vi "handler.vi"(10 "exec queue":refnum<queue>, 11 "connection":refnum<k5>) -> ()   [LabVIEW 2013]
uses:
  worker package.ctl
  application request.ctl
  begin request role.ctl
  record header.ctl
  record types.ctl
  end request body.ctl
  end request protocol status.ctl
  begin request body.ctl
  parse record header.vi
  parse count.vi
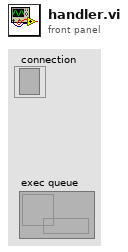
[diagram p1: front panel]
types:
  T1 = typedef "record types.ctl" = enum8{"Error", "Begin Request", "Abort Request", "End Request", "Parameters", "Standard Input", "Standard Output", "Standard Error", "Data", "Get Values", "Get Values Result", "Unknown Type"}
  T2 = typedef "record header.ctl" = cluster{"version":u8, "type":T1, "request id":u16, "content length":u16, "padding length":u8, "reserved":u8}
  T3 = typedef "end request protocol status.ctl" = enum8{"complete", "cant mpx connection", "overloaded", "unknown role"}
  T4 = typedef "end request body.ctl" = cluster{"application status":u32, "protocol status":T3, "reserved 1":u8, "reserved 2":u8, "reserved 3":u8}
  T5 = typedef "begin request body.ctl" = cluster{"role":u16, "flags":u8, "reserved 1":u8, "reserved 2":u8, "reserved 3":u8, "reserved 4":u8, "reserved 5":u8}
  T6 = typedef "application request.ctl" = cluster{"request id":u16, "role":T7, "standard input":string, "data":string, "dictionary":variant, "close after response":bool}
  T7 = typedef "begin request role.ctl" = enum16{"none", "Responder", "Authorizer", "Filter"}
  T8 = typedef "worker package.ctl" = cluster{"TCP Connection":refnum<k5>, "application request":T6}
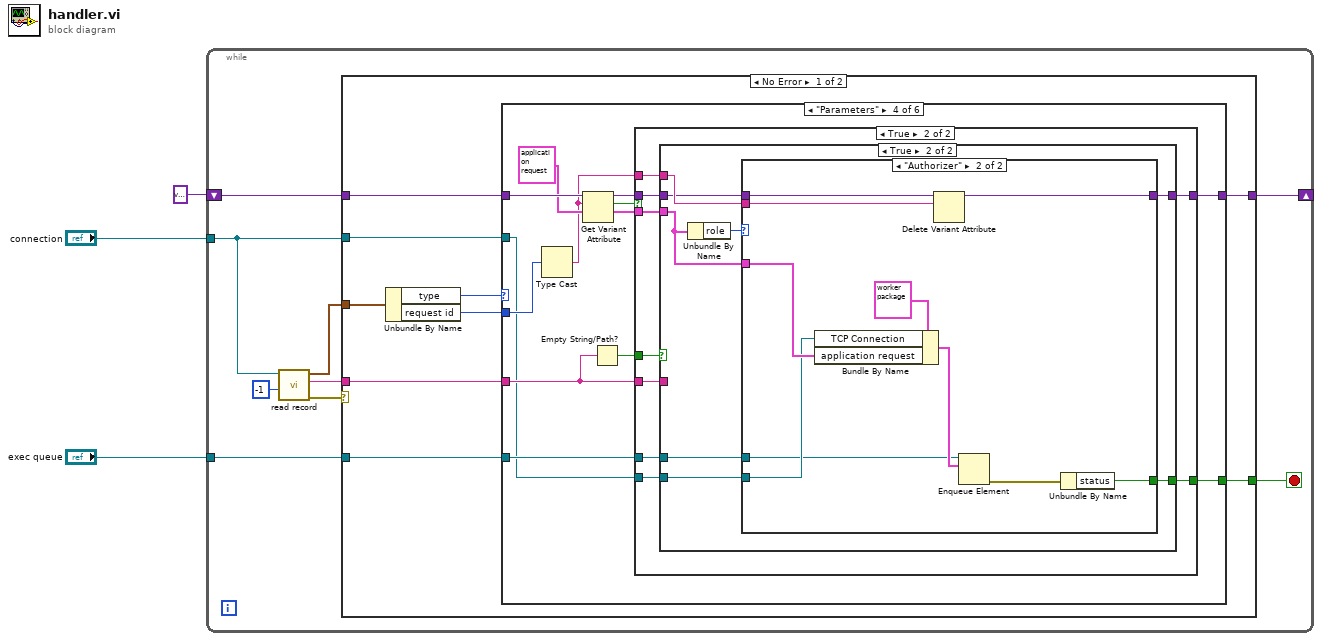
[diagram p0: block diagram]
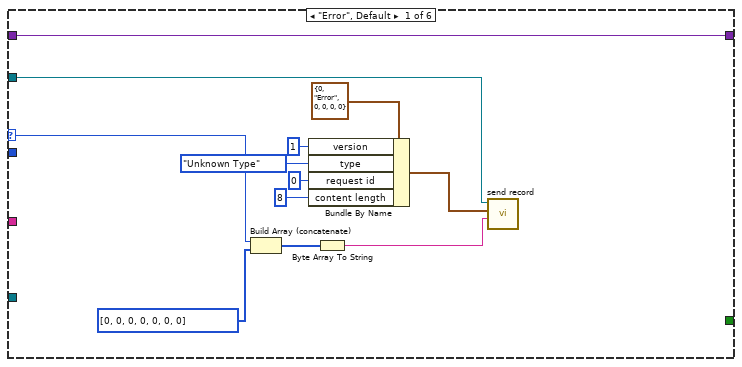
[diagram p2: hidden frame]
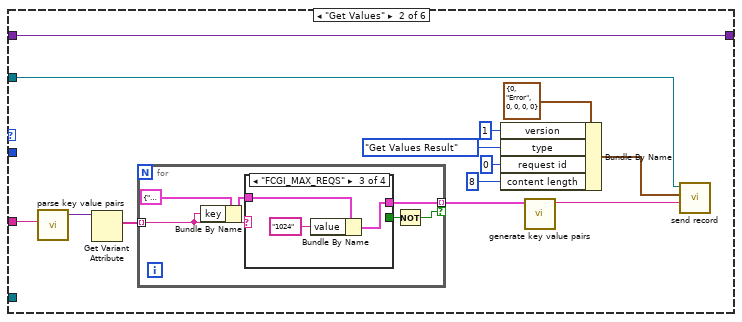
[diagram p3: hidden frame]
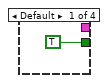
[diagram p4: hidden frame]
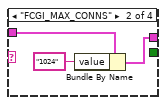
[diagram p5: hidden frame]
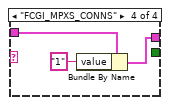
[diagram p6: hidden frame]
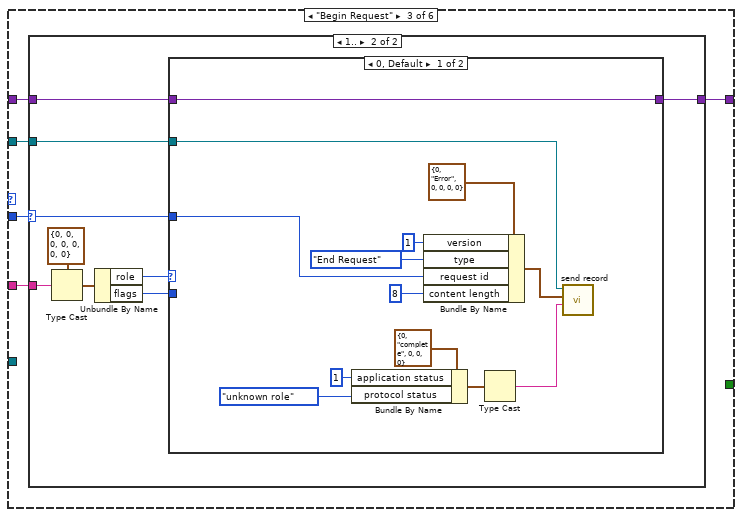
[diagram p7: hidden frame]
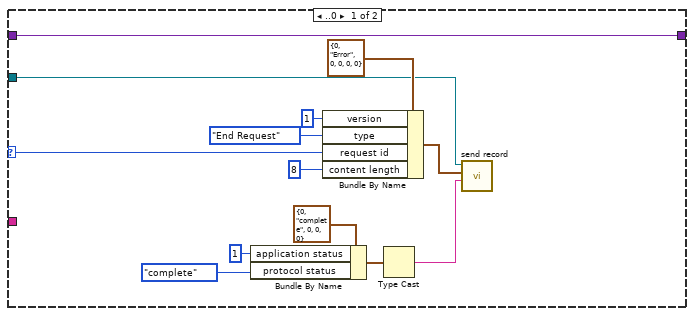
[diagram p8: hidden frame]
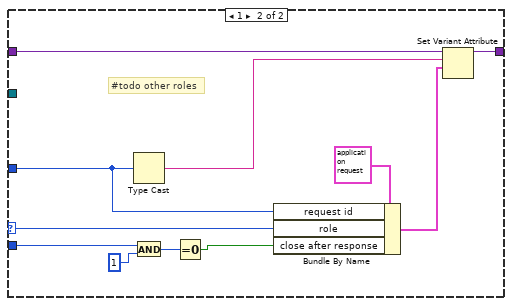
[diagram p9: hidden frame]
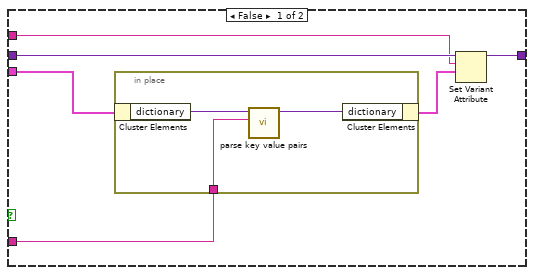
[diagram p11: hidden frame]
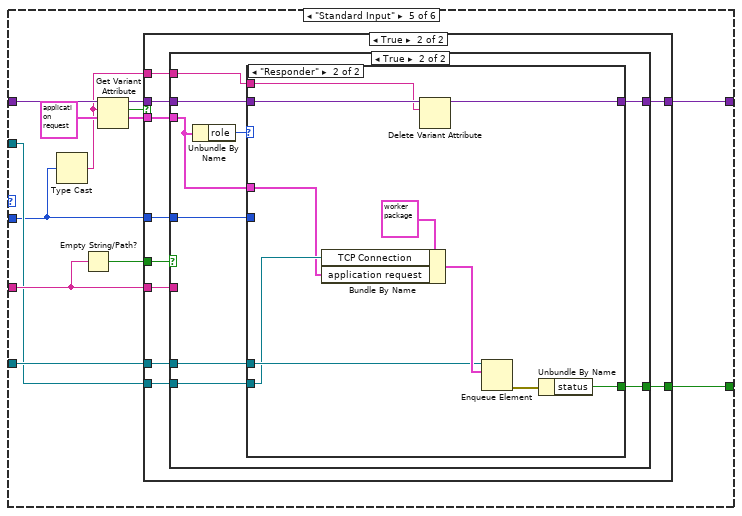
[diagram p13: hidden frame]
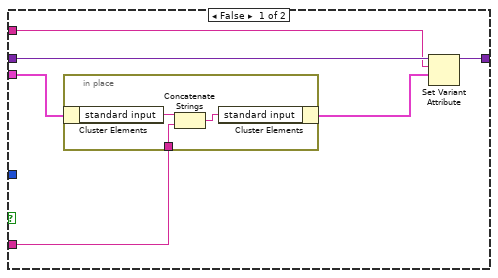
[diagram p15: hidden frame]
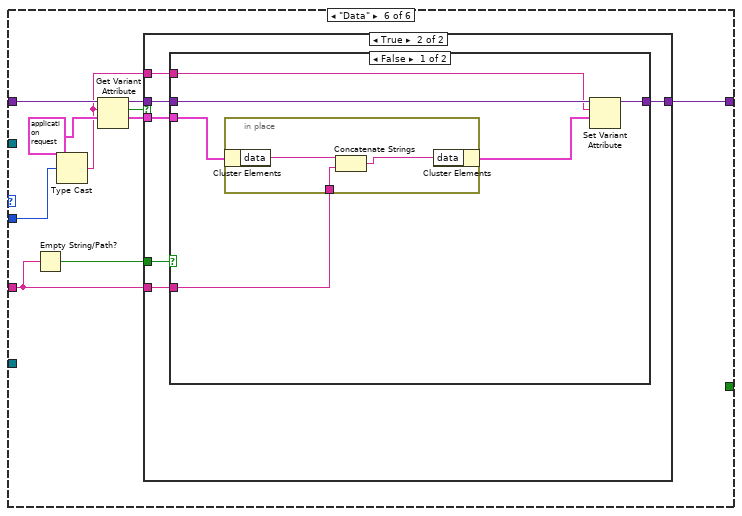
[diagram p17: hidden frame]
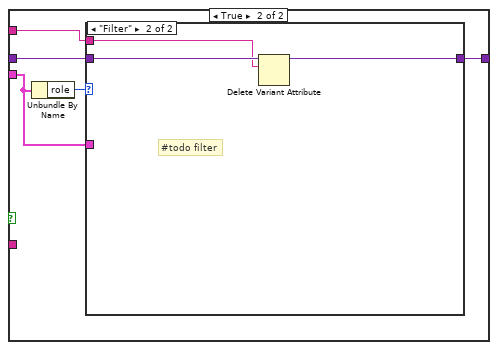
[diagram p19: hidden frame]
diagram:
  n1 = while {
    tunnel: "connection" -> [w6]
    shift-right: [w7] -> _
    shift-left: variant -> [w8]
    tunnel: "exec queue" -> [w4]
    stop <- w5 stop-if-true
    n2 = call "read record.vi"("timeout ms (-1)"=-1, "connection"=w6) -> ("error out"=w11:errorcluster, "data"=w9:string, "header"=w10:T2)  [unwired: 6 in, 1 out]
    n3 = case shown="No Error" w11 {
      tunnel: w10 -> [w21 _]
      tunnel: w9 -> [w15 _]
      tunnel: w8 -> [w19 w254]
      tunnel: [w18 w254] -> w7
      tunnel: w6 -> [w17 _]
      tunnel: [w13 TRUE] -> w5
      tunnel: w4 -> [w14 _]
      frame No Error {
        n4 = Unbundle By Name(w21) -> ("type"=w20:T1, "request id"=w16:u16)
        n5 = case shown="\"Parameters\"" w20 {
          selector: w20 -> [w25 _ _ _ _ _]
          tunnel: w19 -> [w33 w46 w67 w126 w177 w227]
          tunnel: [w33 w46 w65 w125 w176 w226] -> w18
          tunnel: w17 -> [w27 w40 w63 w114 w166 _]
          tunnel: w16 -> [_ _ w64 w124 w165 w225]
          tunnel: w15 -> [_ w36 w66 w123 w175 w224]
          tunnel: w14 -> [_ _ _ w116 w168 _]
          tunnel: [_ _ _ w115 w167 _] -> w13
          frame "Error", Default {
            n6 = Build Array (concatenate)(w25, u8[] [0, 0, 0, 0, 0, 0, 0]) -> (w24:u8[])
            n7 = Bundle By Name(cluster=T2 {"version"=0, "type"=enum."Error", "request id"=0, "content length"=0, "padding length"=0, "reserved"=0} ("header"), "version"=u8 1, "type"=record_types."Unknown Type", "request id"=u16 0, "content length"=u16 8) -> (w26:T2)
            n8 = Byte Array To String(unsigned byte array=w24) -> (string=w23:string)
            n9 = call "send record.vi"("data"=w23, "header"=w26, "connection"=w27) -> ()  [unwired: 8 in, 1 out]
          }
          frame "Get Values" {
            n10 = call "parse key value pairs.vi"("stream"=w36) -> ("dictionary out"=w35:variant)  [unwired: 10 in]
            n11 = Get Variant Attribute(Variant=w35) -> (names=w34:string[])  [unwired: 3 in, 3 out]
            n12 = for {
              tunnel: [w52] -> w37 mode=indexing if=w50
              tunnel: w34 -> [w47] mode=indexing
              n13 = Bundle By Name(cluster=cluster{"key":string, "value":string} {"key"="", "value"=""} ("Cluster"), "key"=w47) -> (w48:cluster{"key":string, "value":string})
              n14 = case shown="\"FCGI_MAX_REQS\"" w47 {
                tunnel: [_ w56 w59 w62] -> w52
                tunnel: [TRUE _ _ _] -> w51
                tunnel: w48 -> [_ w54 w57 w60]
                frame Default {
                }
                frame "FCGI_MAX_CONNS" {
                  n15 = Bundle By Name(cluster=w54, "value"="1024") -> (w56:cluster{"key":string, "value":string})
                }
                frame "FCGI_MAX_REQS" {
                  n16 = Bundle By Name(cluster=w57, "value"="1024") -> (w59:cluster{"key":string, "value":string})
                }
                frame "FCGI_MPXS_CONNS" {
                  n17 = Bundle By Name(cluster=w60, "value"="1") -> (w62:cluster{"key":string, "value":string})
                }
              }
              n18 = Not(x=w51) -> (.not. x?=w50:bool)
            }
            n19 = Bundle By Name(cluster=T2 {"version"=0, "type"=enum."Error", "request id"=0, "content length"=0, "padding length"=0, "reserved"=0} ("header"), "version"=u8 1, "type"=record_types."Get Values Result", "request id"=u16 0, "content length"=u16 8) -> (w39:T2)
            n20 = call "generate key value pairs.vi"("key-value pairs"=w37) -> ("stream"=w38:string)  [unwired: 10 in]
            n21 = call "send record.vi"("data"=w38, "header"=w39, "connection"=w40) -> ()  [unwired: 8 in, 1 out]
          }
          frame "Begin Request" {
            n22 = case shown="1.." w64 {
              selector: w64 -> [w73 w82]
              tunnel: w67 -> [w80 w89]
              tunnel: w66 -> [_ w88]
              tunnel: [w80 w85] -> w65
              tunnel: w63 -> [w74 w81]
              frame ..0 {
                n23 = Bundle By Name(cluster=T4 {"application status"=0, "protocol status"=enum."complete", "reserved 1"=0, "reserved 2"=0, "reserved 3"=0} ("record header"), "application status"=u32 1, "protocol status"=end_request_protocol_status."complete") -> (w70:T4)
                n24 = Bundle By Name(cluster=T2 {"version"=0, "type"=enum."Error", "request id"=0, "content length"=0, "padding length"=0, "reserved"=0} ("header"), "version"=u8 1, "type"=record_types."End Request", "request id"=w73, "content length"=u16 8) -> (w79:T2)
                n25 = Type Cast(x=w70) -> (*(type *) &x=w71:string)  [unwired: 1 in]
                n26 = call "send record.vi"("data"=w71, "header"=w79, "connection"=w74) -> ()  [unwired: 8 in, 1 out]
              }
              frame 1.. {
                n27 = Type Cast(type=T5 {"role"=0, "flags"=0, "reserved 1"=0, "reserved 2"=0, "reserved 3"=0, "reserved 4"=0, "reserved 5"=0} ("record header"), x=w88) -> (*(type *) &x=w86:T5)
                n28 = Unbundle By Name(w86) -> ("role"=w83:u16, "flags"=w84:u8)
                n29 = case shown="0, Default" w83 {
                  selector: w83 -> [_ w105]
                  tunnel: w89 -> [w102 w113]
                  tunnel: [w102 w111] -> w85
                  tunnel: w84 -> [_ w109]
                  tunnel: w82 -> [w90 w103]
                  tunnel: w81 -> [w91 _]
                  frame 0, Default {
                    n30 = Bundle By Name(cluster=T4 {"application status"=0, "protocol status"=enum."complete", "reserved 1"=0, "reserved 2"=0, "reserved 3"=0} ("record header"), "application status"=u32 1, "protocol status"=end_request_protocol_status."unknown role") -> (w99:T4)
                    n31 = Bundle By Name(cluster=T2 {"version"=0, "type"=enum."Error", "request id"=0, "content length"=0, "padding length"=0, "reserved"=0} ("header"), "version"=u8 1, "type"=record_types."End Request", "request id"=w90, "content length"=u16 8) -> (w92:T2)
                    n32 = Type Cast(x=w99) -> (*(type *) &x=w98:string)  [unwired: 1 in]
                    n33 = call "send record.vi"("data"=w98, "header"=w92, "connection"=w91) -> ()  [unwired: 8 in, 1 out]
                  }
                  frame 1 {
                    # "#todo other roles"
                    n34 = Type Cast(x=w103) -> (*(type *) &x=w104:string)  [unwired: 1 in]
                    n35 = And(x=w109, y=u8 1) -> (x .and. y?=w107:u8)
                    n36 = Equal To 0?(x=w107) -> (x = 0?=w106:bool)
                    n37 = Bundle By Name(cluster=T6 {"request id"=0, "role"=enum."none", "standard input"="", "data"="", "dictionary"=variant(cluster{"key":string, "value":string}[] []), "close after response"=FALSE} ("application request"), "request id"=w103, "role"=w105, "close after response"=w106) -> (w110:T6)
                    n38 = Set Variant Attribute(Variant=w113, name=w104, value=w110) -> (Variant out=w111:variant)  [unwired: 1 in, 2 out]
                  }
                }
              }
            }
          }
          frame "Parameters" {
            n39 = Type Cast(x=w124) -> (*(type *) &x=w118:string)  [unwired: 1 in]
            n40 = Get Variant Attribute(Variant=w126, name=w118, default value (empty Variant)=T6 {"request id"=0, "role"=enum."Responder", "standard input"="", "data"="", "dictionary"=variant(cluster{"key":string, "value":string}[] []), "close after response"=FALSE} ("application request")) -> (duplicate Variant=w122:variant, found=w120:bool, value=w119:T6)  [unwired: 1 in, 1 out]
            n41 = Empty String/Path?(string/path=w123) -> (empty?=w117:bool)
            n42 = case shown="True" w120 {
              tunnel: w122 -> [w127 w136]
              tunnel: [w127 w135] -> w125
              tunnel: w119 -> [_ w132]
              tunnel: w118 -> [_ w134]
              tunnel: w123 -> [_ w133]
              tunnel: w117 -> [_ w131]
              tunnel: w116 -> [_ w130]
              tunnel: [_ w129] -> w115
              tunnel: w114 -> [_ w128]
              frame False {
              }
              frame True {
                n43 = case shown="True" w131 {
                  tunnel: w136 -> [w142 w151]
                  tunnel: [w141 w150] -> w135
                  tunnel: w134 -> [w140 w152]
                  tunnel: w133 -> [w137 _]
                  tunnel: w132 -> [w139 w149]
                  tunnel: w130 -> [_ w148]
                  tunnel: [_ w147] -> w129
                  tunnel: w128 -> [_ w146]
                  frame False {
                    n44 = in-place {
                      in-place-border: w137 -> [w145]
                      n45 = in-place-cluster #1(w139) -> ("dictionary"=w144:variant)
                      n46 = call "parse key value pairs.vi"("stream"=w145, "dictionary in"=w144) -> ("dictionary out"=w143:variant)  [unwired: 9 in]
                      n47 = in-place-cluster #1("dictionary"=w143) -> (w138:T6)
                    }
                    n48 = Set Variant Attribute(Variant=w142, name=w140, value=w138) -> (Variant out=w141:variant)  [unwired: 1 in, 2 out]
                  }
                  frame True {
                    n49 = Unbundle By Name(w149) -> ("role"=w153:T7)
                    n50 = case shown="\"Authorizer\"" w153 {
                      tunnel: w152 -> [_ w162]
                      tunnel: w151 -> [w154 w164]
                      tunnel: [w154 w163] -> w150
                      tunnel: w149 -> [_ w157]
                      tunnel: w148 -> [_ w155]
                      tunnel: [_ w161] -> w147
                      tunnel: w146 -> [_ w156]
                      frame "none", Default {
                      }
                      frame "Authorizer" {
                        n51 = Bundle By Name(cluster=T8 {"TCP Connection"=refnum, "application request"={"request id"=0, "role"=enum."none", "standard input"="", "data"="", "dictionary"=variant(cluster{"key":string, "value":string}[] []), "close after response"=FALSE}} ("request package"), "TCP Connection"=w156, "application request"=w157) -> (w159:T8)
                        n52 = Delete Variant Attribute(6:w162, 7:w164) -> (3:w163:variant)  [unwired: 1 in, 2 out]
                        n53 = Enqueue Element(queue=w155, element=w159) -> (error out=w158:errorcluster)  [unwired: 2 in, 2 out]
                        n54 = Unbundle By Name(w158) -> ("status"=w161:bool)
                      }
                    }
                  }
                }
              }
            }
          }
          frame "Standard Input" {
            n55 = Type Cast(x=w165) -> (*(type *) &x=w170:string)  [unwired: 1 in]
            n56 = Empty String/Path?(string/path=w175) -> (empty?=w169:bool)
            n57 = Get Variant Attribute(Variant=w177, name=w170, default value (empty Variant)=T6 {"request id"=0, "role"=enum."Responder", "standard input"="", "data"="", "dictionary"=variant(cluster{"key":string, "value":string}[] []), "close after response"=FALSE} ("application request")) -> (duplicate Variant=w174:variant, found=w172:bool, value=w171:T6)  [unwired: 1 in, 1 out]
            n58 = case shown="True" w172 {
              tunnel: w174 -> [w178 w188]
              tunnel: [w178 w187] -> w176
              tunnel: w171 -> [_ w185]
              tunnel: w170 -> [_ w186]
              tunnel: w175 -> [_ w184]
              tunnel: w169 -> [_ w183]
              tunnel: w168 -> [_ w182]
              tunnel: [_ w181] -> w167
              tunnel: w166 -> [_ w180]
              tunnel: w165 -> [_ w179]
              frame False {
              }
              frame True {
                n59 = case shown="True" w183 {
                  tunnel: w188 -> [w194 w204]
                  tunnel: [w193 w205] -> w187
                  tunnel: w186 -> [w192 w203]
                  tunnel: w185 -> [w191 w202]
                  tunnel: w184 -> [w189 _]
                  tunnel: w182 -> [_ w201]
                  tunnel: [_ w200] -> w181
                  tunnel: w180 -> [_ w199]
                  tunnel: w179 -> [_ w198]
                  frame False {
                    n60 = in-place {
                      in-place-border: w189 -> [w195]
                      n61 = in-place-cluster #2(w191) -> ("standard input"=w197:string)
                      n62 = Concatenate Strings(w197, w195) -> (w196:string)
                      n63 = in-place-cluster #2("standard input"=w196) -> (w190:T6)
                    }
                    n64 = Set Variant Attribute(Variant=w194, name=w192, value=w190) -> (Variant out=w193:variant)  [unwired: 1 in, 2 out]
                  }
                  frame True {
                    n65 = Unbundle By Name(w202) -> ("role"=w206:T7)
                    n66 = case shown="\"Responder\"" w206 {
                      tunnel: [w207 w216] -> w205
                      tunnel: w204 -> [w207 w217]
                      tunnel: w203 -> [_ w215]
                      tunnel: w202 -> [_ w208]
                      tunnel: w201 -> [_ w210]
                      tunnel: [_ w214] -> w200
                      tunnel: w199 -> [_ w209]
                      tunnel: w198 -> [_ _]
                      frame Default {
                      }
                      frame "Responder" {
                        n67 = Bundle By Name(cluster=T8 {"TCP Connection"=refnum, "application request"={"request id"=0, "role"=enum."none", "standard input"="", "data"="", "dictionary"=variant(cluster{"key":string, "value":string}[] []), "close after response"=FALSE}} ("request package"), "TCP Connection"=w209, "application request"=w208) -> (w213:T8)
                        n68 = Delete Variant Attribute(6:w215, 7:w217) -> (3:w216:variant)  [unwired: 1 in, 2 out]
                        n69 = Enqueue Element(queue=w210, element=w213) -> (error out=w211:errorcluster)  [unwired: 2 in, 2 out]
                        n70 = Unbundle By Name(w211) -> ("status"=w214:bool)
                      }
                    }
                  }
                }
              }
            }
          }
          frame "Data" {
            n71 = Empty String/Path?(string/path=w224) -> (empty?=w218:bool)
            n72 = Type Cast(x=w225) -> (*(type *) &x=w219:string)  [unwired: 1 in]
            n73 = Get Variant Attribute(Variant=w227, name=w219, default value (empty Variant)=T6 {"request id"=0, "role"=enum."Responder", "standard input"="", "data"="", "dictionary"=variant(cluster{"key":string, "value":string}[] []), "close after response"=FALSE} ("application request")) -> (duplicate Variant=w223:variant, found=w221:bool, value=w220:T6)  [unwired: 1 in, 1 out]
            n74 = case shown="True" w221 {
              tunnel: w223 -> [w228 w234]
              tunnel: [w228 w233] -> w226
              tunnel: w220 -> [_ w231]
              tunnel: w219 -> [_ w232]
              tunnel: w224 -> [_ w230]
              tunnel: w218 -> [_ w229]
              frame False {
              }
              frame True {
                n75 = case shown="False" w229 {
                  tunnel: w234 -> [w240 w246]
                  tunnel: [w239 w247] -> w233
                  tunnel: w232 -> [w238 w245]
                  tunnel: w231 -> [w237 w244]
                  tunnel: w230 -> [w235 _]
                  frame False {
                    n76 = in-place {
                      in-place-border: w235 -> [w241]
                      n77 = in-place-cluster #3(w237) -> ("data"=w243:string)
                      n78 = Concatenate Strings(w243, w241) -> (w242:string)
                      n79 = in-place-cluster #3("data"=w242) -> (w236:T6)
                    }
                    n80 = Set Variant Attribute(Variant=w240, name=w238, value=w236) -> (Variant out=w239:variant)  [unwired: 1 in, 2 out]
                  }
                  frame True {
                    n81 = Unbundle By Name(w244) -> ("role"=w248:T7)
                    n82 = case shown="\"Filter\"" w248 {
                      tunnel: [w249 w251] -> w247
                      tunnel: w246 -> [w249 w252]
                      tunnel: w245 -> [_ w250]
                      tunnel: w244 -> [_ _]
                      frame Default {
                      }
                      frame "Filter" {
                        # "#todo filter"
                        n83 = Delete Variant Attribute(6:w250, 7:w252) -> (3:w251:variant)  [unwired: 1 in, 2 out]
                      }
                    }
                  }
                }
              }
            }
          }
        }
      }
      frame Error {
      }
    }
  }
